vi "74HC151的功能测试.vi"(0 "D 0":bool, 1 "D 1":bool, 2 "D 2":bool, 3 "D 3":bool, 4 "D 4":bool, 5 "D 5":bool, 6 "D 6":bool, 7 "D 7":bool, 8 "A0":bool, 10 "A1":bool, 11 "EN":bool, 12 "A2":bool) -> (23 "Y":bool)   [LabVIEW 2018]
panel:
  in  "结束":bool
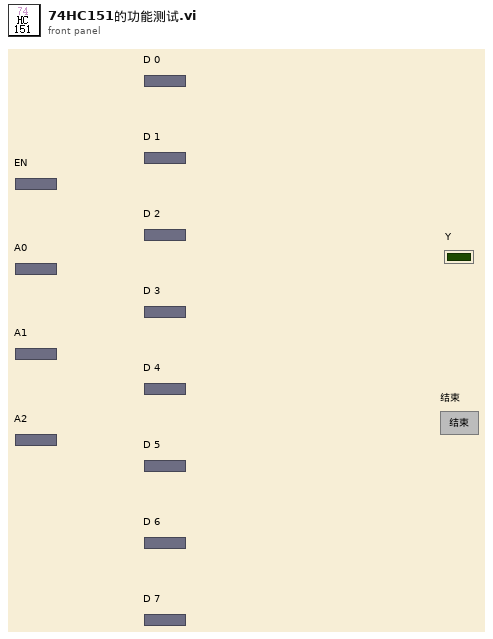
[diagram p1: front panel]
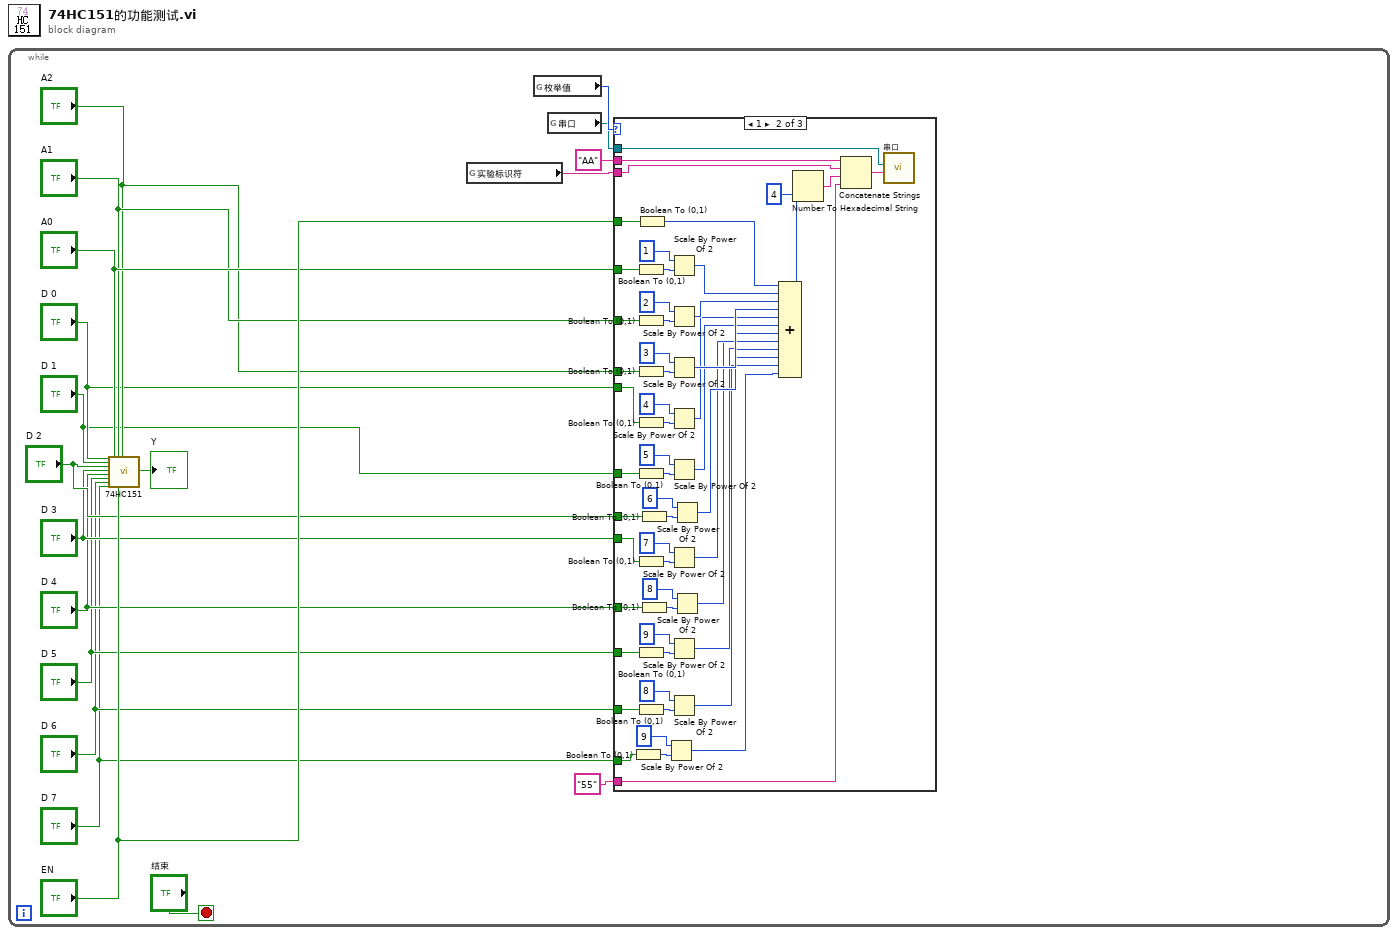
[diagram p0: block diagram]
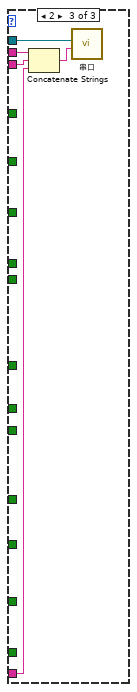
[diagram p3: hidden frame]
diagram:
  n1 = while {
    stop <- "结束" stop-if-true
    n2 = call "74HC151.vi"("D 0"="D 0", "D 1"="D 1", "D 2"="D 2", "D 3"="D 3", "D 4"="D 4", "D 5"="D 5", "D 6"="D 6", "D 7"="D 7", "A0"="A0", "A1"="A1", "EN"="EN", "A2"="A2") -> ("布尔"=→"Y":bool)  [unwired: 15 in]
    n3 = global read "全局变量.vi" "实验标识符"() -> (w16:string)
    n4 = global read "全局变量.vi" "枚举值"() -> (w18:i8)
    n5 = global read "全局变量.vi" "串口"() -> (w17:refnum<visa-resource-name>)
    n6 = case shown="1" w18 {
      tunnel: w17 -> [_ w68 w76]
      tunnel: w16 -> [_ w67 w77]
      tunnel: "55" -> [_ w66 w74]
      tunnel: "AA" -> [_ w65 w75]
      tunnel: "EN" -> [_ w31 _]
      tunnel: "A0" -> [_ w30 _]
      tunnel: "A1" -> [_ w29 _]
      tunnel: "A2" -> [_ w28 _]
      tunnel: "D 0" -> [_ w27 _]
      tunnel: "D 1" -> [_ w26 _]
      tunnel: "D 2" -> [_ w25 _]
      tunnel: "D 3" -> [_ w24 _]
      tunnel: "D 4" -> [_ w23 _]
      tunnel: "D 5" -> [_ w22 _]
      tunnel: "D 6" -> [_ w21 _]
      tunnel: "D 7" -> [_ w20 _]
      frame 0, Default {
      }
      frame 1 {
        n7 = Boolean To (0,1)(Boolean=w20) -> (0, 1=w39:i16)
        n8 = Boolean To (0,1)(Boolean=w30) -> (0, 1=w70:i16)
        n9 = Boolean To (0,1)(Boolean=w29) -> (0, 1=w60:i16)
        n10 = Boolean To (0,1)(Boolean=w28) -> (0, 1=w58:i16)
        n11 = Boolean To (0,1)(Boolean=w27) -> (0, 1=w56:i16)
        n12 = Boolean To (0,1)(Boolean=w26) -> (0, 1=w54:i16)
        n13 = Boolean To (0,1)(Boolean=w24) -> (0, 1=w47:i16)
        n14 = Boolean To (0,1)(Boolean=w22) -> (0, 1=w43:i16)
        n15 = Boolean To (0,1)(Boolean=w21) -> (0, 1=w41:i16)
        n16 = Boolean To (0,1)(Boolean=w31) -> (0, 1=w72:i16)
        n17 = Boolean To (0,1)(Boolean=w25) -> (0, 1=w49:i16)
        n18 = Boolean To (0,1)(Boolean=w23) -> (0, 1=w45:i16)
        n19 = Scale By Power Of 2(n=9, x=w39) -> (x*2^n=w32:i16)
        n20 = Scale By Power Of 2(n=1, x=w70) -> (x*2^n=w71:i16)
        n21 = Scale By Power Of 2(n=2, x=w60) -> (x*2^n=w61:i16)
        n22 = Scale By Power Of 2(n=3, x=w58) -> (x*2^n=w52:i16)
        n23 = Scale By Power Of 2(n=4, x=w56) -> (x*2^n=w51:i16)
        n24 = Scale By Power Of 2(n=5, x=w54) -> (x*2^n=w50:i16)
        n25 = Scale By Power Of 2(n=7, x=w47) -> (x*2^n=w36:i16)
        n26 = Scale By Power Of 2(n=9, x=w43) -> (x*2^n=w34:i16)
        n27 = Scale By Power Of 2(n=8, x=w41) -> (x*2^n=w33:i16)
        n28 = Scale By Power Of 2(n=6, x=w49) -> (x*2^n=w37:i16)
        n29 = Scale By Power Of 2(n=8, x=w45) -> (x*2^n=w35:i16)
        n30 = Compound Arithmetic op=ADD ("复合运算")(w72, w71, w61, w52, w51, w50, w37, w36, w35, w34, w33, w32) -> (w64:i16)
        n31 = Number To Hexadecimal String(1:4, 2:w64) -> (0:w62:string)
        n32 = Concatenate Strings(w65, w67, w62, w66) -> (w73:string)
        n33 = call "串口.vi"("字符串"=w73, "VISA resource name"=w68) -> ()  [unwired: 10 in]
      }
      frame 2 {
        n34 = Concatenate Strings(w75, w77, w74) -> (w78:string)
        n35 = call "串口.vi"("字符串"=w78, "VISA resource name"=w76) -> ()  [unwired: 10 in]
      }
    }
  }
